vi "OAT Polar Phase Value Conversion.vi"(9 "channel settings":T1 {"probe angle [deg]" max=360 step=1; "shaft rotating direction" items=["CCW", "CW"]}, 11 "phases in":dbl[](array[numeric]) format="%.2f") -> (3 "phases out":dbl[](array[numeric]) format="%.2f")   [LabVIEW 2017]
uses:
  <vilib>/Analysis/NI_AALPro.lvlib
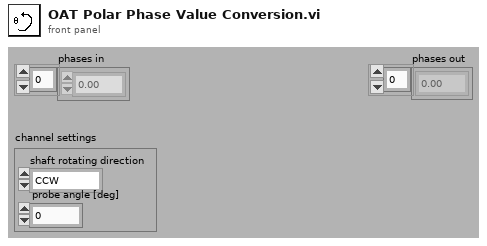
[diagram p1: front panel]
types:
  T1 = cluster{"shaft rotating direction":u16, "probe angle [deg]":u16}
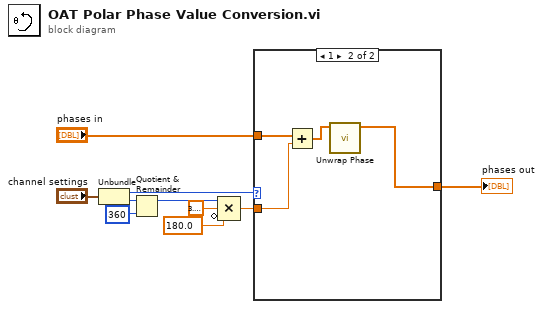
[diagram p0: block diagram]
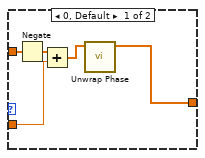
[diagram p2: hidden frame]
diagram:
  n1 = Unbundle("channel settings") -> ("shaft rotating direction"=w7:u16, "probe angle [deg]"=w4:u16)
  n2 = Quotient & Remainder(x=w4, y=u16 360) -> (x-y*floor(x/y)=w2:u16)  [unwired: 1 out]
  n3 = Compound Arithmetic op=MULTIPLY(w2, 3.141592653589793, invert 180.0 ("value")) -> (w6:dbl)
  n4 = case shown="1" w7 {
    tunnel: [w13 w17] -> w10
    tunnel: "phases in" -> [w14 w19]
    tunnel: w6 -> [w11 w16]
    frame 0, Default {
      n5 = Negate(x=w14) -> (-x=w12:dbl[])
      n6 = Add(x=w12, y=w11) -> (x+y=w15:dbl[])
      n7 = call <vilib>:"Unwrap Phase.vi"("Phase"=w15) -> ("Unwrapped Phase"=w13:dbl[])  [unwired: 9 in, 1 out]
    }
    frame 1 {
      n8 = Add(x=w19, y=w16) -> (x+y=w18:dbl[])
      n9 = call <vilib>:"Unwrap Phase.vi"("Phase"=w18) -> ("Unwrapped Phase"=w17:dbl[])  [unwired: 9 in, 1 out]
    }
  }
  "phases out" <- w10
